vi "MOKE_Teperature and FIeld Sweep_1022D.vi"() -> ()   [LabVIEW 2022 SP3]
uses:
  <vilib>/Analysis/baseanly.llb/Mean (DBL).vi
  <vilib>/Utility/file.llb/Write Delimited Spreadsheet (string).vi
  <vilib>/Utility/file.llb/Write Delimited Spreadsheet (DBL).vi
  <vilib>/Analysis/NI_AALBase.lvlib
panel:
  in  "Read Status":bool
  in  "Wait for position/focus check every (Oe)":i32
  out "Rh1 B/A v F":cluster{dbl[], dbl[]}(graph)
  out "Temperature Status":i32(ring) items=["TemperatureUnknown"=0, "Stable"=1, "Tracking"=2, "Near"=5, "Chasing"=6, "Filling"=7, "Standby"=10, "Disabled"=13, "ImpedanceNotFunction"=14, "TempFailure"=15]
  out "Field Status":i32(ring) items=["MagnetUnknown"=0, "StablePersistent"=1, "WarmingSwitch"=2, "CoolingSwitch"=3, "StableDriven"=4, "Iterating"=5, "Charging"=6, "Discharging"=7, "CurrentError"=8, "MagnetFailure"=15]
  out "Field":dbl
  out "Temperature":dbl
  in  "Initialize":bool
  in  "System Stablization (s)":dbl=0.1 format="%#_13g"
  in  "Low Value (Oe)":dbl=-30000.0
  in  "High Value (Oe)":dbl=30000.0
  in  "Sweep Field Approach":i32(ring) items=["Linear", "NoOvershoot", "Oscillate"]
  in  "Sweep F Rate (Oe/s)":dbl=200.0 format="%#_13g"
  in  "Sweep F mode":i32(ring) items=["Persistent", "Driven"]
  in  "Set Fixed T":dbl=2.0
  in  "Fixed Temperature Approach":i32(ring)=1 items=["FastSettle", "NoOvershoot"]
  in  "FIxed T  Rate (K/min)":dbl=20.0
  out "PhaseA-F":cluster{dbl[], dbl[]}(graph)
  out "RA-F":cluster{dbl[], dbl[]}(graph)
  out "Phaseh1B-F":cluster{dbl[], dbl[]}(graph)
  out "Rh1B-F":cluster{dbl[], dbl[]}(graph)
  out "phase B 2":dbl
  in  "Phase B 2":u16(ring)=3 items=["X", "Y", "R", "Theta", "Frequency", "Noise", "Xh1", "Yh1", "Rh1", "Theta h1", "Xh2", "Yh2", "Rh2", "Theta h2"]
  out "phase A 2":dbl
  in  "Phase A 2":u16(ring)=3 items=["X", "Y", "R", "Theta", "Frequency", "Noise", "Xh1", "Yh1", "Rh1", "Theta h1", "Xh2", "Yh2", "Rh2", "Theta h2"]
  out "para1 Measurement (mV) 2":dbl=1.49013e-07
  in  "F Clear Plot A":bool
  in  "Parameter A 2":u16(ring)=2 items=["X", "Y", "R", "Theta", "Frequency", "Noise", "Xh1", "Yh1", "Rh1", "Theta h1", "Xh2", "Yh2", "Rh2", "Theta h2"]
  out "para2 Measurement (uV) 2":dbl=1.49013e-07
  in  "F Clear Plot B":bool
  in  "Parameter B 2":u16(ring)=2 items=["X", "Y", "R", "Theta", "Frequency", "Noise", "Xh1", "Yh1", "Rh1", "Theta h1", "Xh2", "Yh2", "Rh2", "Theta h2"]
  out "Field Setting":dbl format="%#_13g"
  out "Fixed Temperature":dbl
  out "Measured Field":dbl
  out "Field Status":i32(ring) items=["MagnetUnknown"=0, "StablePersistent"=1, "WarmingSwitch"=2, "CoolingSwitch"=3, "StableDriven"=4, "Iterating"=5, "Charging"=6, "Discharging"=7, "CurrentError"=8, "MagnetFailure"=15]
  out "Temperature Status":i32(ring) items=["TemperatureUnknown"=0, "Stable"=1, "Tracking"=2, "Near"=5, "Chasing"=6, "Filling"=7, "Standby"=10, "Disabled"=13, "ImpedanceNotFunction"=14, "TempFailure"=15]
  out "Measuring F":bool
  in  "Step(Oe)":i32=2000
  out "F loop run":i32
  out "Temperature Status":i32(ring) items=["TemperatureUnknown"=0, "Stable"=1, "Tracking"=2, "Near"=5, "Chasing"=6, "Filling"=7, "Standby"=10, "Disabled"=13, "ImpedanceNotFunction"=14, "TempFailure"=15]
  out "Field Status":i32(ring) items=["MagnetUnknown"=0, "StablePersistent"=1, "WarmingSwitch"=2, "CoolingSwitch"=3, "StableDriven"=4, "Iterating"=5, "Charging"=6, "Discharging"=7, "CurrentError"=8, "MagnetFailure"=15]
  out "Fixed Field":dbl
  out "Measured Temperature":dbl
  in  "Delay(T/F)":dbl=5.0
  in  "Set FIxed F (Oe)":dbl format="%#_13g"
  in  "Fixed Field Approach":i32(ring) items=["Linear", "NoOvershoot", "Oscillate"]
  in  "FIxed F Rate (Oe/s)":dbl=100.0 format="%#_13g"
  in  "Fixed F mode":i32(ring) items=["Persistent", "Driven"]
  in  "Sweep Temperature Approach":i32(ring)=1 items=["FastSettle", "NoOvershoot"]
  in  "Sweep T  Rate (K/min)":dbl=10.0
  in  "Sweep T/F":bool
  in  "Remote":bool=TRUE
  in  "IP Address":string="169.254.170.239"
  out "Measuring T":bool
  in  "A Sine Output Amplitude (V)":sgl=0.1
  in  "path (folder + filename)":string="C:\\Users\\Public\\OneDrive\\Desktop\\MOKE program\\sweep files"
  in  "LOCKIN address":refnum<visa-resource-name>="COM3"
  out "PhaseA-T":cluster{dbl[], dbl[]}(graph)
  out "RA-T":cluster{dbl[], dbl[]}(graph)
  out "Phaseh1-T":cluster{dbl[], dbl[]}(graph)
  out "Rh1B-T":cluster{dbl[], dbl[]}(graph)
  out "phase B":dbl
  in  "Phase B":u16(ring)=9 items=["X", "Y", "R", "Theta", "Frequency", "Noise", "Xh1", "Yh1", "Rh1", "Theta h1", "Xh2", "Yh2", "Rh2", "Theta h2"]
  out "phase A":dbl
  in  "Phase A":u16(ring)=3 items=["X", "Y", "R", "Theta", "Frequency", "Noise", "Xh1", "Yh1", "Rh1", "Theta h1", "Xh2", "Yh2", "Rh2", "Theta h2"]
  out "para1 Measurement (mV)":dbl=1.49013e-07
  in  "T Clear Plot A":bool
  in  "Parameter A":u16(ring)=2 items=["X", "Y", "R", "Theta", "Frequency", "Noise", "Xh1", "Yh1", "Rh1", "Theta h1", "Xh2", "Yh2", "Rh2", "Theta h2"]
  out "para2 Measurement (uV)":dbl=1.49013e-07
  in  "T Clear Plot B":bool
  in  "Parameter B":u16(ring)=8 items=["X", "Y", "R", "Theta", "Frequency", "Noise", "Xh1", "Yh1", "Rh1", "Theta h1", "Xh2", "Yh2", "Rh2", "Theta h2"]
  out "Temperature Setting":dbl format="%#_13g"
  in  "Save data or not":bool=TRUE
  in  "Step(K)":i32=10
  out "T loop run":i32
  in  "B frequency":dbl=267.7 format="%#_13g"
  in  "B Input Connection (0: Single-Ended)":u16(ring)=1 items=["Single-Ended Voltage", "Differential Voltage", "1 MOhm Current Gain", "100 MOhm Current Gain"]
  in  "B harmonic 1":u8=2
  in  "B harmonic 2":u8=3
  in  "B reference Manual Phase":dbl=-59.75
  in  "auto phase B":bool=TRUE
  in  "B Sample time (s)":dbl=0.001 min=0.001 max=100.0 step=0.001
  in  "B Sensitivity":u16(ring)=20 items=["1 nV/fA", "2 nV/fA", "5 nV/fA", "10 nV/fA", "20 nV/fA", "50 nV/fA", "100 nV/fA", "200 nV/fA", "500 nV/fA", "1 uV/pA", "2 uV/pA", "5 uV/pA", "10 uV/pA", "20 uV/pA", "50 uV/pA", "100 uV/pA", "200 uV/pA", "500 uV/pA", "1 mV/nA", "2 mV/nA", "5 mV/nA", "10 mV/nA", "20 mV/nA", "50 mV/nA", "100 mV/nA", "200 mV/nA", "500 mV/nA", "1 V/uA"]
  in  "Enable Sync Filter B (open when f<200Hz)":bool
  in  "B Time Constant":u8(ring)=9 items=["10 us", "30 us", "100 us", "300 us", "1 ms", "3 ms", "10 ms", "30 ms", "100 ms", "300 ms", "1 s", "3 s", "10 s", "30 s", "100 s", "300 s", "1 ks", "3 ks"]
  in  "B Reference Source":u8(ring) items=["External", "Internal", "Internal Sweep", "Channel-A"]
  in  "B Low Pass Filter Slope":u8(ring)=2 items=["6 dB/oct", "12 dB/oct", "18 db/oct", "24 dB/oct"]
  in  "A frequency":dbl=267.7 format="%#_13g"
  in  "A Input Connection (0: Single-Ended)":u16(ring)=1 items=["Single-Ended Voltage", "Differential Voltage", "1 MOhm Current Gain", "100 MOhm Current Gain"]
  in  "A harmonic 1":u8=2
  in  "A harmonic 2":u8=3
  in  "A reference Manual Phase":dbl=-59.75
  in  "auto phase A":bool=TRUE
  in  "A Reference Source":u8(ring)=1 items=["External", "Internal", "Internal Sweep"]
  in  "A Sample time (s)":dbl=0.001 min=0.001 max=100.0 step=0.001
  in  "A Time Constant":u8(ring)=9 items=["10 us", "30 us", "100 us", "300 us", "1 ms", "3 ms", "10 ms", "30 ms", "100 ms", "300 ms", "1 s", "3 s", "10 s", "30 s", "100 s", "300 s", "1 ks", "3 ks"]
  in  "Enable Sync Filter A (open when f<200Hz)":bool
  in  "A Sensitivity":u16(ring)=20 items=["1 nV/fA", "2 nV/fA", "5 nV/fA", "10 nV/fA", "20 nV/fA", "50 nV/fA", "100 nV/fA", "200 nV/fA", "500 nV/fA", "1 uV/pA", "2 uV/pA", "5 uV/pA", "10 uV/pA", "20 uV/pA", "50 uV/pA", "100 uV/pA", "200 uV/pA", "500 uV/pA", "1 mV/nA", "2 mV/nA", "5 mV/nA", "10 mV/nA", "20 mV/nA", "50 mV/nA", "100 mV/nA", "200 mV/nA", "500 mV/nA", "1 V/uA"]
  in  "A Low Pass Filter Slope":u8(ring)=2 items=["6 dB/oct", "12 dB/oct", "18 db/oct", "24 dB/oct"]
  in  "stabilization(S)":dbl=0.1 format="%#_13g"
  in  "High Value (K)":dbl=300.0
  in  "Low Value (K)":dbl=2.0
  in  "loop #":i32=1
  # "Status"
  # "opticool ip addresse: 169.254.170.239"
  # "Lock-in Setting"
  # "Channel A"
  # "Channel B"
  # "Sweep F Mesurement"
  # "Temprature and Field Setting"
  # "Sweep T Mesurement"
  # "Sweep F"
  # "Sweep T"
  # "0 for no checks"
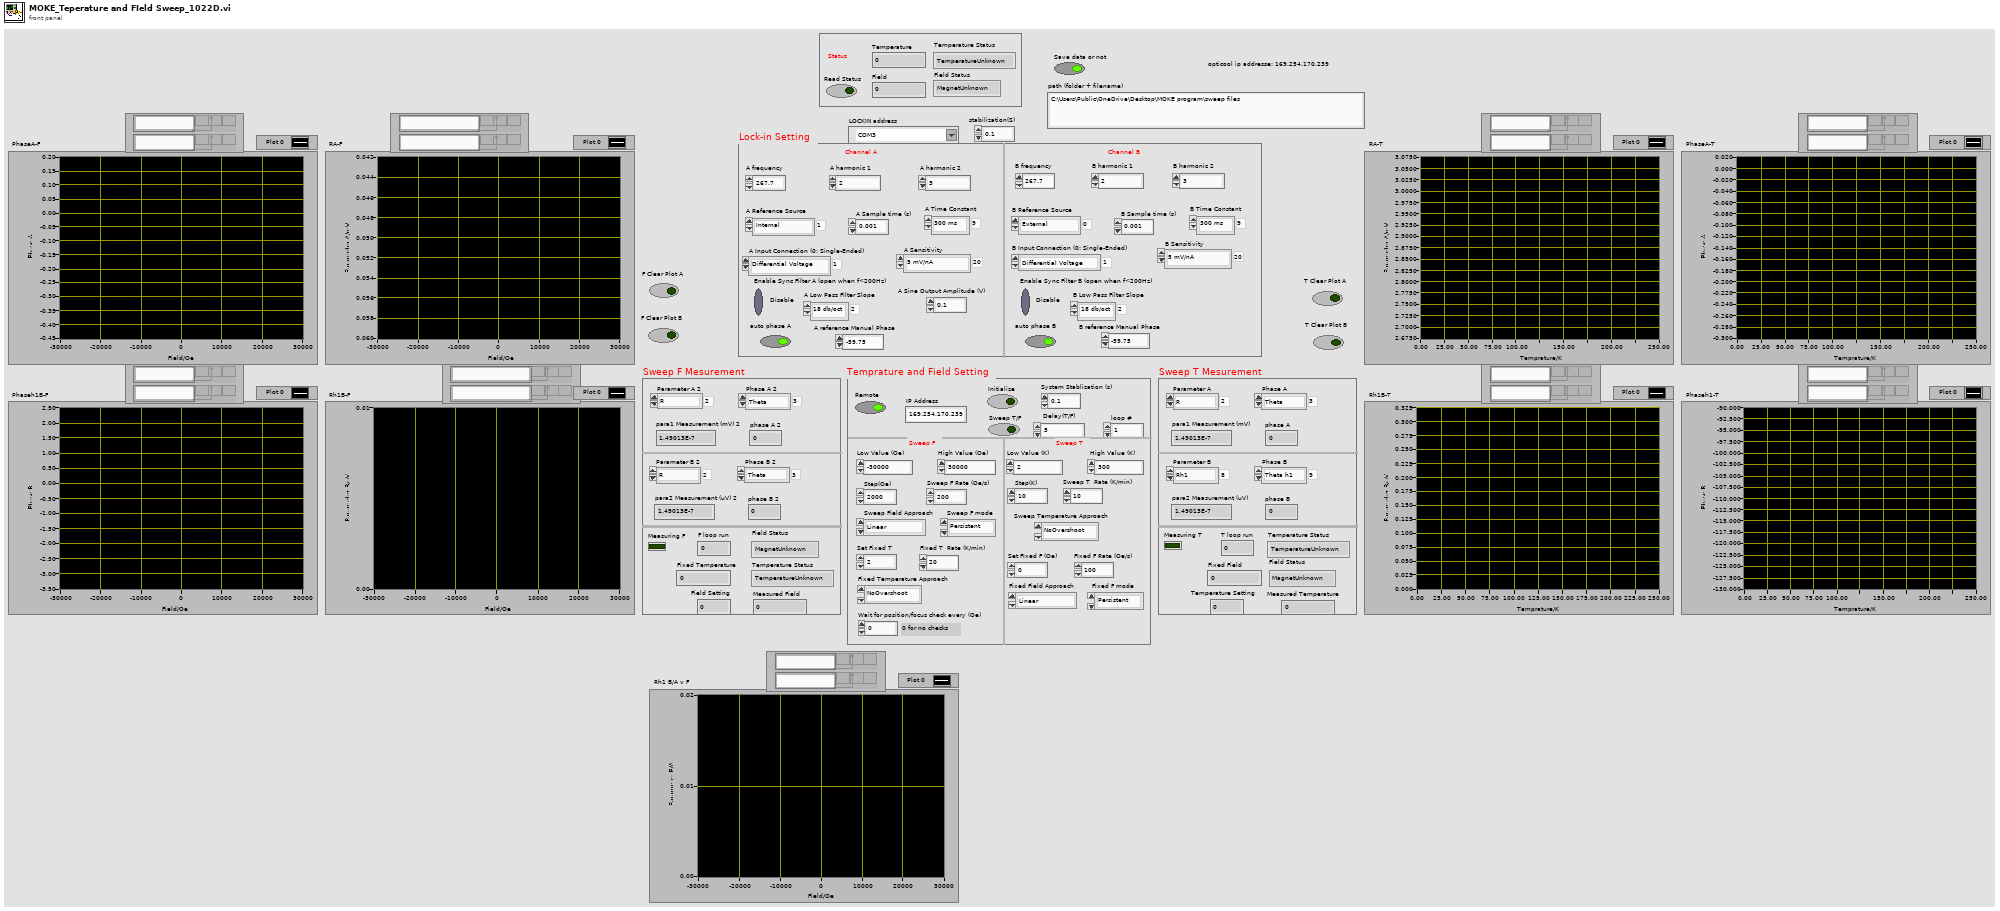
[diagram p1: front panel]
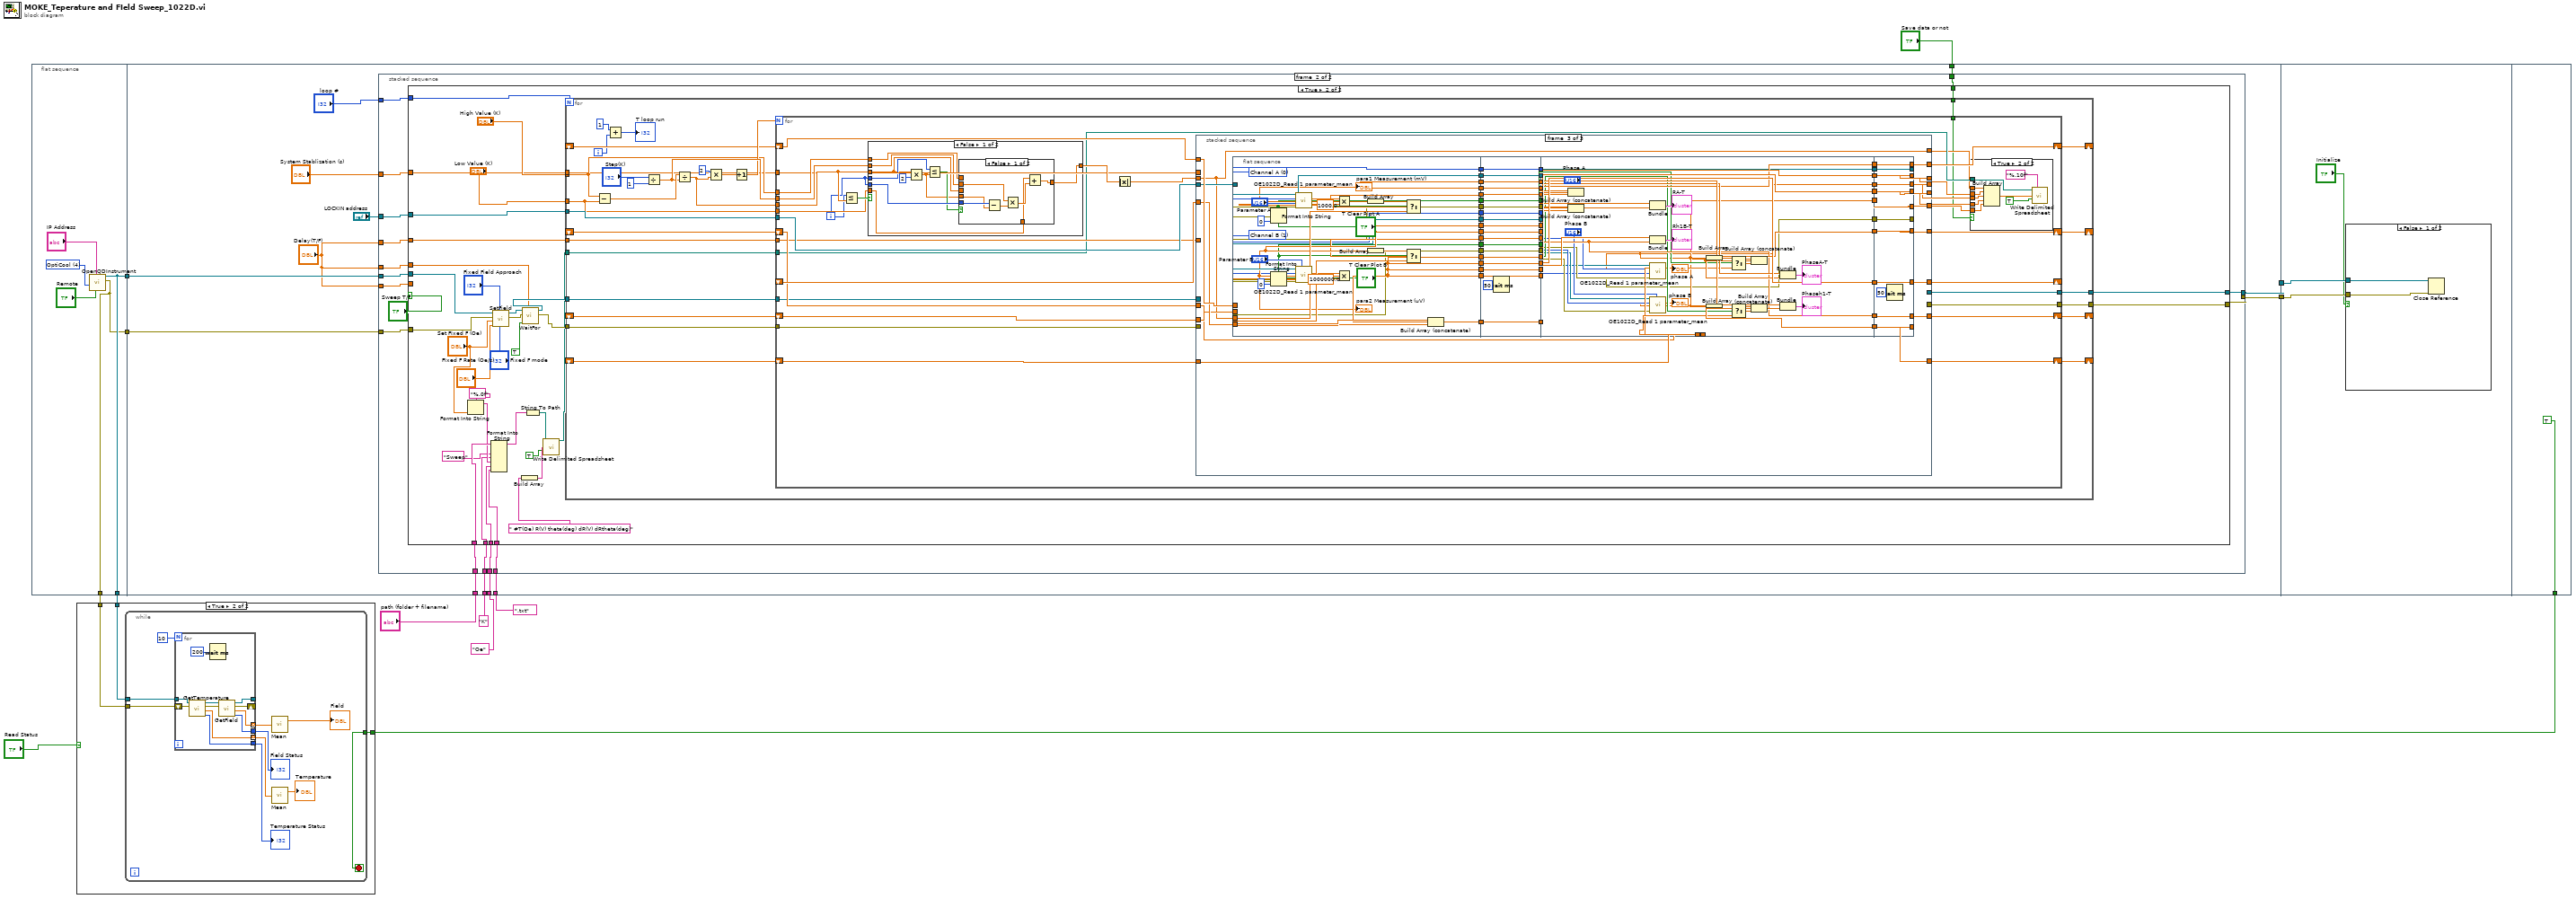
[diagram p0: block diagram]
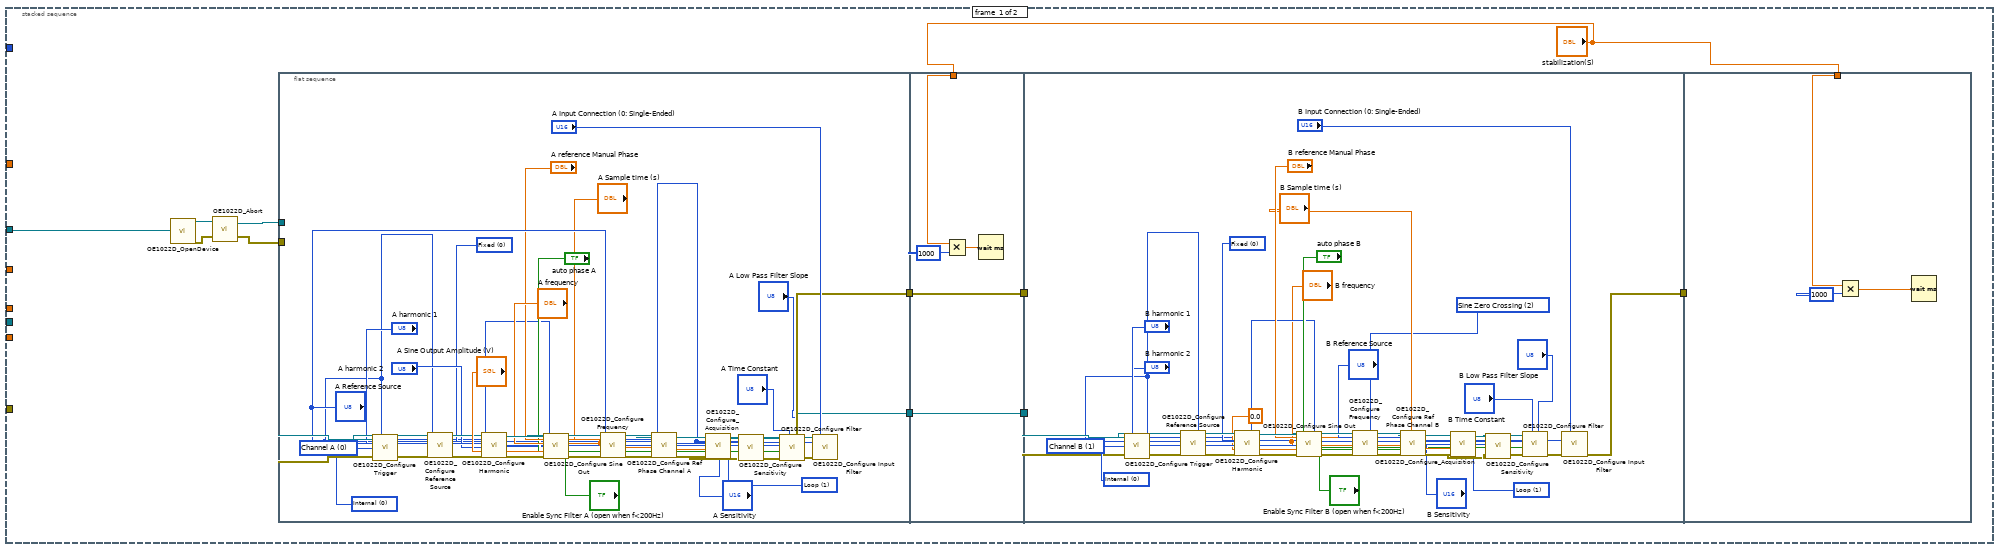
[diagram p3: hidden frame]
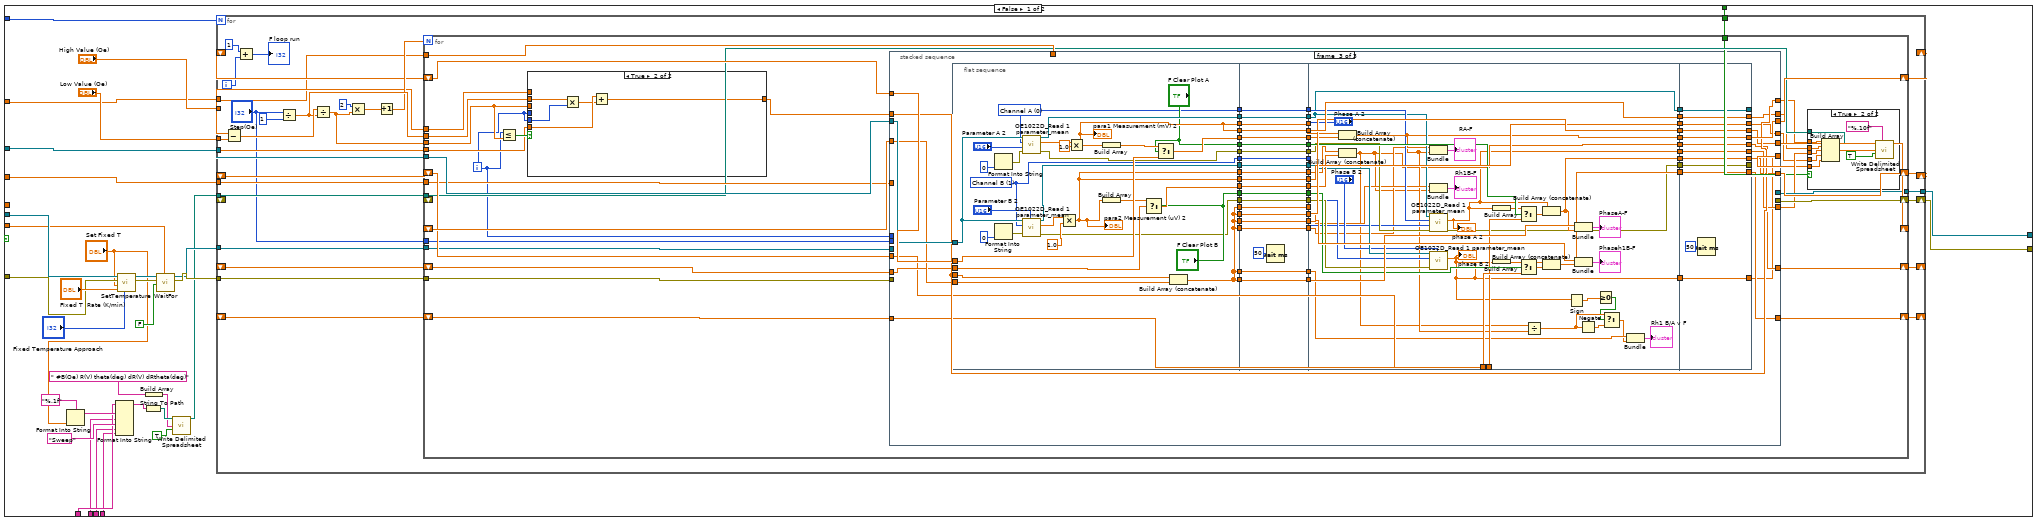
[diagram p4: hidden frame]
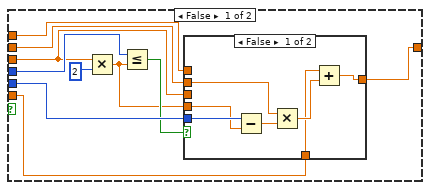
[diagram p6: hidden frame]
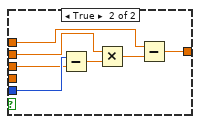
[diagram p7: hidden frame]
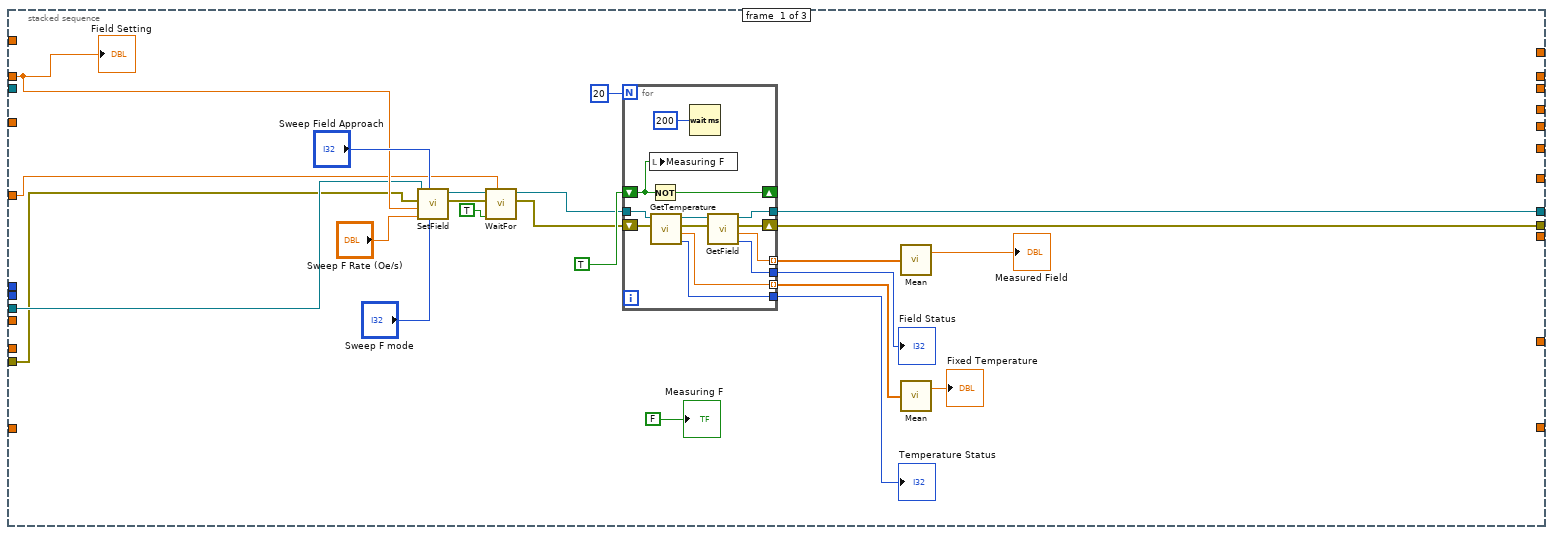
[diagram p8: hidden frame]
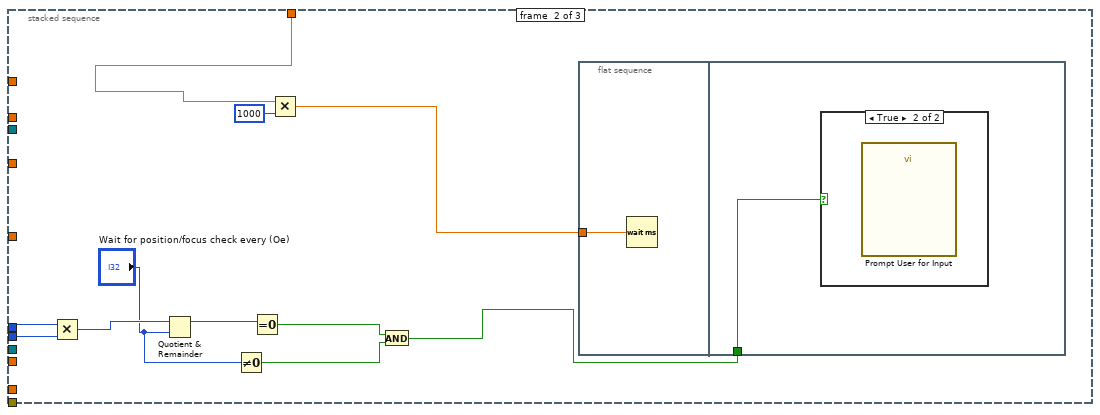
[diagram p9: hidden frame]
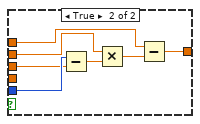
[diagram p12: hidden frame]
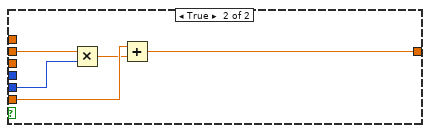
[diagram p13: hidden frame]
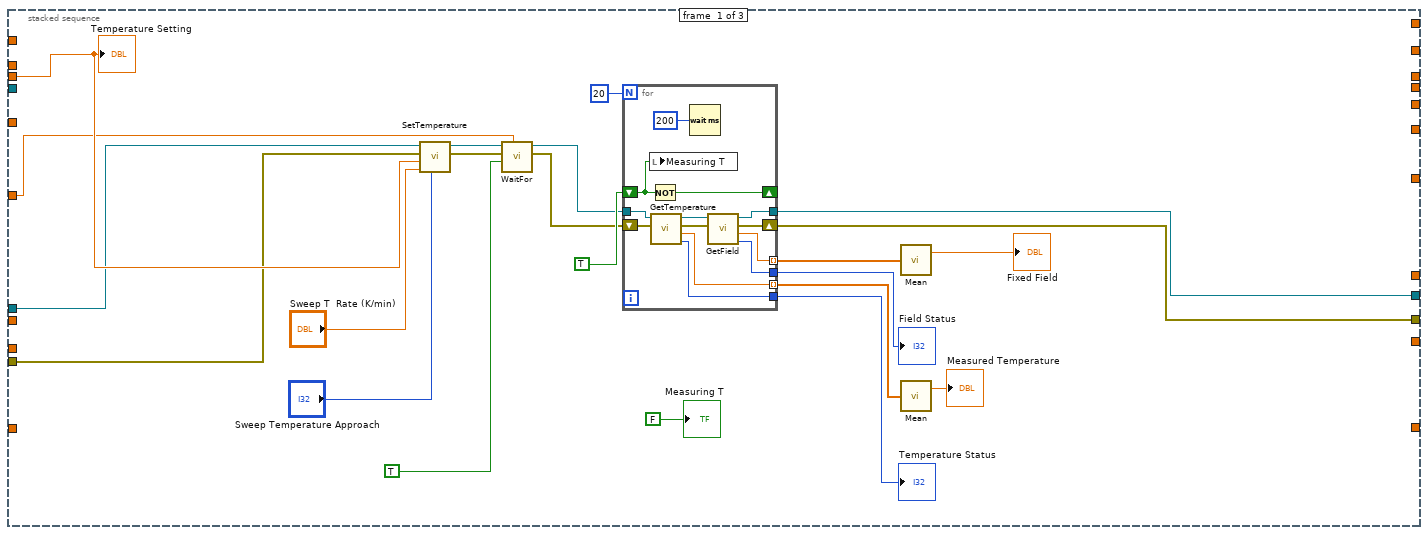
[diagram p14: hidden frame]
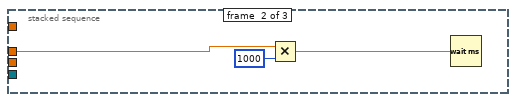
[diagram p15: hidden frame]
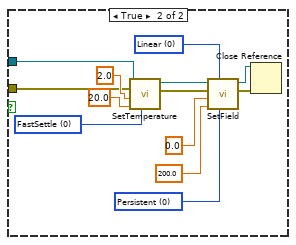
[diagram p16: hidden frame]
diagram:
  n1 = flat-sequence {
    tunnel: [w15] -> w13
    tunnel: [w14] -> w12
    tunnel: [w15] -> w5
    tunnel: [w14] -> w4
    tunnel: w13 -> [w29]
    tunnel: w12 -> [w28]
    tunnel: "path (folder + filename)" -> [w26]
    tunnel: "Oe" -> [w25]
    tunnel: "K" -> [w24]
    tunnel: ".txt" -> [w23]
    tunnel: [w21] -> w7
    tunnel: [w20] -> w6
    tunnel: "Save data or not" -> [w19]
    tunnel: w7 -> [w840]
    tunnel: w6 -> [w839]
    tunnel: [TRUE] -> w2
    frame #0 {
      w16 = 4 items=["PPMS", "VersaLab", "DynaCool", "SVSM", "OptiCool"] ("InstrumentType")
      n2 = call "OpenQDInstrument.vi"("Remote"="Remote", "IP Address"="IP Address", "InstrumentType"=w16) -> ("error out"=w14:errorcluster, "Instrument Ref"=w15:refnum<k24>)  [unwired: 5 in]
    }
    frame #1 {
      n3 = stacked-sequence {
        tunnel: "LOCKIN address" -> [w34 w143]
        tunnel: "loop #" -> [_ w142]
        tunnel: w29 -> [_ w140]
        tunnel: w28 -> [_ w139]
        tunnel: "Delay(T/F)" -> [_ w138]
        tunnel: "Delay(T/F)" -> [_ w137]
        tunnel: "Delay(T/F)" -> [_ w136]
        tunnel: w26 -> [_ w135]
        tunnel: w25 -> [_ w134]
        tunnel: w24 -> [_ w133]
        tunnel: w23 -> [_ w132]
        tunnel: "System Stablization (s)" -> [_ w131]
        tunnel: [_ w130] -> w21
        tunnel: [_ w129] -> w20
        tunnel: w19 -> [_ w128]
        frame #0 {
          n4 = call "OE1022D_OpenDevice.vi"("VISA resource name"=w34) -> ("VISA资源名称输出"=w33:refnum<visa-resource-name>, "错误输出"=w35:errorcluster)  [unwired: 17 in]
          n5 = call "OE1022D_Abort.vi"("error in (no error)"=w35, "VISA resource name"=w33) -> ("error out"=w40:errorcluster, "VISA resource name out"=w41:refnum<visa-resource-name>)
          n6 = flat-sequence {
            tunnel: w41 -> [w81]
            tunnel: [w69] -> w39
            tunnel: w40 -> [w80]
            tunnel: [w57] -> w37
            tunnel: w39 -> [w86]
            tunnel: [w86] -> w38
            tunnel: w37 -> [w85]
            tunnel: [w85] -> w36
            tunnel: "stabilization(S)" -> [w82]
            tunnel: w38 -> [w107]
            tunnel: [w106] -> w42
            tunnel: w36 -> [w105]
            tunnel: w42 -> [_]
            tunnel: "stabilization(S)" -> [w125]
            frame #0 {
              w43 = u8 1 items=["Single", "Loop"] ("Sample Mode (Single/Loop)")
              w56 = u8 0 items=["Fixed", "Linear", "Log"] ("SineOut Mode")
              w58 = u16 0 items=["Internal", "External"] ("Trigger Source (0: Internal)")
              w47 = u8 0 items=["Channel A", "Channel B"] ("OE1022D A/B")
              n7 = call "OE1022D_Configure Trigger.vi"("Trigger Source (0: Internal)"=w58, "error in (no error)   2"=w80, "OE1022D A/B"=w47, "VISA resource name   2"=w81) -> ("error out   2"=w74:errorcluster, "VISA resource name out   2"=w75:refnum<visa-resource-name>)
              n8 = call "OE1022D_Configure Reference Source.vi"("VISA resource name"=w75, "OE1022D A/B"=w47, "Reference Source"="A Reference Source", "error in (no error)"=w74) -> ("VISA resource name out"=w73:refnum<visa-resource-name>, "error out"=w71:errorcluster)  [unwired: 14 in]
              n9 = call "OE1022D_Configure Harmonic.vi"("VISA resource name"=w73, "OE1022D A/B"=w47, "Harmonic 1"="A harmonic 1", "Harmonic 2"="A harmonic 2", "error in (no error)"=w71) -> ("VISA resource name out"=w72:refnum<visa-resource-name>, "error out"=w70:errorcluster)  [unwired: 13 in]
              n10 = call "OE1022D_Configure Sine Out.vi"("VISA resource name"=w72, "SineOut Mode"=w56, "OE1022D A/B"=w47, "Sine Output Amplitude (V)"="A Sine Output Amplitude (V)", "error in (no error)"=w70) -> ("VISA resource name out"=w78:refnum<visa-resource-name>, "error out"=w77:errorcluster)  [unwired: 9 in]
              n11 = call "OE1022D_Configure Frequency.vi"("VISA resource name"=w78, "OE1022D A/B"=w47, "Internal Frequency(Hz)"="A frequency", "error in (no error)"=w77) -> ("VISA resource name out"=w68:refnum<visa-resource-name>, "error out"=w65:errorcluster)  [unwired: 14 in]
              n12 = call "OE1022D_Configure Ref Phase Channel A.vi"("VISA resource name"=w68, "Reference Source"="A Reference Source", "Internal Frequency(Hz)"="A frequency", "Auto Phase (T: Enabled)"="auto phase A", "error in (no error)"=w65, "Manual Phase  (degree)"="A reference Manual Phase") -> ("VISA resource name out"=w67:refnum<visa-resource-name>, "error out"=w66:errorcluster)  [unwired: 12 in]
              n13 = call "OE1022D_Configure_Acquisition.vi"("VISA resource name"=w67, "OE1022D A/B"=w47, "Sample time (s)"="A Sample time (s)", "error in (no error)"=w66, "Sample Mode (Single/Loop)"=w43) -> ("VISA resource name out"=w50:refnum<visa-resource-name>, "error out"=w49:errorcluster)  [unwired: 3 in]
              n14 = call "OE1022D_Configure Sensitivity.vi"("VISA resource name"=w50, "OE1022D A/B"=w47, "Sensitivity"="A Sensitivity", "error in (no error)"=w49) -> ("VISA resource name out"=w54:refnum<visa-resource-name>, "error out"=w53:errorcluster)  [unwired: 14 in]
              n15 = call "OE1022D_Configure Filter.vi"("Low Pass Filter Slope (1: 12dB/oct)"="A Low Pass Filter Slope", "Time Constant (8: 100ms)"="A Time Constant", "error in (no error)"=w53, "Enable Sync Filter (F: Disable)"="Enable Sync Filter A (open when f<200Hz)", "OE1022D A/B"=w47, "VISA resource name"=w54) -> ("error out"=w51:errorcluster, "VISA resource name out"=w52:refnum<visa-resource-name>)  [unwired: 4 in]
              n16 = call "OE1022D_Configure Input Filter.vi"("VISA resource name"=w52, "Input Source"="A Input Connection (0: Single-Ended)", "OE1022D A/B"=w47, "error in (no error)"=w51) -> ("VISA resource name out"=w57:refnum<visa-resource-name>, "error out"=w69:errorcluster)  [unwired: 10 in]
            }
            frame #1 {
              n17 = Multiply(x=w82, y=1000) -> (x*y=w84:dbl)
              n18 = Wait (ms)(milliseconds to wait=w84) -> ()  [unwired: 1 out]
            }
            frame #2 {
              w87 = u8 1 items=["Single", "Loop"] ("Sample Mode (Single/Loop)")
              w89 = u8 2 items=["TTL Pos", "TTL Neg", "Sine Zero Crossing"] ("External Ref Trigger")
              w102 = u8 0 items=["Fixed", "Linear", "Log"] ("SineOut Mode")
              w108 = u16 0 items=["Internal", "External"] ("Trigger Source (0: Internal)")
              w94 = u8 1 items=["Channel A", "Channel B"] ("OE1022D A/B")
              n19 = call "OE1022D_Configure Trigger.vi"("Trigger Source (0: Internal)"=w108, "error in (no error)   2"=w107, "OE1022D A/B"=w94, "VISA resource name   2"=w105) -> ("error out   2"=w120:errorcluster, "VISA resource name out   2"=w121:refnum<visa-resource-name>)
              n20 = call "OE1022D_Configure Reference Source.vi"("VISA resource name"=w121, "OE1022D A/B"=w94, "error in (no error)"=w120) -> ("VISA resource name out"=w119:refnum<visa-resource-name>, "error out"=w117:errorcluster)  [unwired: 15 in]
              n21 = call "OE1022D_Configure Harmonic.vi"("VISA resource name"=w119, "OE1022D A/B"=w94, "Harmonic 1"="B harmonic 1", "Harmonic 2"="B harmonic 2", "error in (no error)"=w117) -> ("VISA resource name out"=w118:refnum<visa-resource-name>, "error out"=w116:errorcluster)  [unwired: 13 in]
              n22 = call "OE1022D_Configure Sine Out.vi"("VISA resource name"=w118, "SineOut Mode"=w102, "OE1022D A/B"=w94, "Sine Output Amplitude (V)"=sgl 0.0, "error in (no error)"=w116) -> ("VISA resource name out"=w123:refnum<visa-resource-name>, "error out"=w122:errorcluster)  [unwired: 9 in]
              n23 = call "OE1022D_Configure Frequency.vi"("VISA resource name"=w123, "OE1022D A/B"=w94, "Internal Frequency(Hz)"="B frequency", "error in (no error)"=w122) -> ("VISA resource name out"=w115:refnum<visa-resource-name>, "error out"=w112:errorcluster)  [unwired: 14 in]
              n24 = call "OE1022D_Configure Ref Phase Channel B.vi"("VISA resource name"=w115, "Reference Source"="B Reference Source", "External Ref Trigger"=w89, "Internal Frequency(Hz)"="B frequency", "Auto Phase (T: Enabled)"="auto phase B", "error in (no error)"=w112, "Manual Phase  (degree)"="B reference Manual Phase") -> ("VISA resource name out"=w114:refnum<visa-resource-name>, "error out"=w113:errorcluster)  [unwired: 11 in]
              n25 = call "OE1022D_Configure_Acquisition.vi"("VISA resource name"=w114, "OE1022D A/B"=w94, "Sample time (s)"="B Sample time (s)", "error in (no error)"=w113, "Sample Mode (Single/Loop)"=w87) -> ("VISA resource name out"=w95:refnum<visa-resource-name>, "error out"=w96:errorcluster)  [unwired: 3 in]
              n26 = call "OE1022D_Configure Sensitivity.vi"("VISA resource name"=w95, "OE1022D A/B"=w94, "Sensitivity"="B Sensitivity", "error in (no error)"=w96) -> ("VISA resource name out"=w99:refnum<visa-resource-name>, "error out"=w98:errorcluster)  [unwired: 14 in]
              n27 = call "OE1022D_Configure Filter.vi"("Low Pass Filter Slope (1: 12dB/oct)"="B Low Pass Filter Slope", "Time Constant (8: 100ms)"="B Time Constant", "error in (no error)"=w98, "Enable Sync Filter (F: Disable)"="Enable Sync Filter B (open when f<200Hz)", "OE1022D A/B"=w94, "VISA resource name"=w99) -> ("error out"=w97:errorcluster)  [unwired: 4 in, 1 out]
              n28 = call "OE1022D_Configure Input Filter.vi"("Input Source"="B Input Connection (0: Single-Ended)", "OE1022D A/B"=w94, "error in (no error)"=w97) -> ("error out"=w106:errorcluster)  [unwired: 11 in, 1 out]
            }
            frame #3 {
              n29 = Multiply(x=w125, y=1000) -> (x*y=w127:dbl)
              n30 = Wait (ms)(milliseconds to wait=w127) -> ()  [unwired: 1 out]
            }
          }
        }
        frame #1 {
          n31 = case shown="True" "Sweep T/F" {
            tunnel: w143 -> [w175 w534]
            tunnel: w142 -> [w176 w533]
            tunnel: w140 -> [w167 w529]
            tunnel: w139 -> [w168 w528]
            tunnel: w138 -> [_ w522]
            tunnel: w137 -> [w174 w521]
            tunnel: w136 -> [w166 _]
            tunnel: w135 -> [w158 w517]
            tunnel: w134 -> [w157 w513]
            tunnel: w133 -> [w156 w514]
            tunnel: w132 -> [w155 w512]
            tunnel: w131 -> [w152 w509]
            tunnel: [w151 w508] -> w130
            tunnel: [w150 w507] -> w129
            tunnel: w128 -> [w149 w506]
            frame False {
              n32 = Format Into String(format string="%.1f", "Set Fixed T") -> (resulting string=w160:string)  [unwired: 2 in, 1 out]
              n33 = Format Into String(initial string=w158, w160, w156, "Sweep", w157, w155) -> (resulting string=w161:string)  [unwired: 2 in, 1 out]
              n34 = call "SetTemperature.vi"("Approach"="Fixed Temperature Approach", "Rate"="FIxed T  Rate (K/min)", "Temperature"="Set Fixed T", "error in (no error)"=w168, "Instrument Ref In"=w167) -> ("error out"=w169:errorcluster, "Instrument Ref Out"=w170:refnum<k24>)  [unwired: 2 in, 1 out]
              n35 = String To Path(string=w161) -> (path=w148:path)
              n36 = Build Array(" #B(Oe) R(V) theta(deg) dR(V) dRtheta(deg)") -> (w146:string[])
              n37 = call "WaitFor.vi"("Delay"=w166, "Wait For Temperature"=FALSE ("WaitForTemperature"), "error in (no error)"=w169, "Instrument Ref In"=w170) -> ("error out"=w165:errorcluster, "Instrument Ref Out"=w164:refnum<k24>)  [unwired: 6 in]
              n38 = call-poly <vilib>:"Write Delimited Spreadsheet.vi"("file path (dialog if empty)"=w148, "1D data"=w146, "append to file? (new file:F)"=TRUE) -> ("new file path (Not A Path if cancelled)"=w145:path)  [unwired: 11 in, 1 out]
              n39 = for {
                N: w176 -> [_]
                tunnel: w175 -> [w206]
                tunnel: "Low Value (Oe)" -> [w201]
                tunnel: "High Value (Oe)" -> [w191]
                tunnel: w145 -> [w200]
                shift-right: [w196] -> _
                shift-left: _ -> [w195]
                shift-right: [w190] -> _
                shift-left: _ -> [w189]
                shift-right: [w188] -> _
                shift-left: _ -> [w187]
                shift-right: [w186] -> _
                shift-left: _ -> [w185]
                tunnel: w164 -> [w184]
                tunnel: w165 -> [w183]
                tunnel: w174 -> [w182]
                tunnel: w152 -> [w181]
                shift-right: [w180] -> w151
                shift-left: _ -> [_]
                tunnel: [w179] -> w150
                tunnel: w149 -> [w178]
                i -> [w193]
                n40 = Subtract(x=w191, y=w201) -> (x-y=w203:dbl)
                n41 = Add(x=1, y=w193) -> (x+y=→"F loop run":i32)
                n42 = Divide(x="Step(Oe)", y=1) -> (x/y=w202:dbl)
                n43 = Divide(x=w203, y=w202) -> (x/y=w199:dbl)
                n44 = Multiply(x=2, y=w199) -> (x*y=w198:dbl)
                n45 = Increment(x=w198) -> (x+1=w197:dbl)
                n46 = for {
                  N: w197 -> [_]
                  tunnel: w206 -> [w238]
                  tunnel: w202 -> [w234]
                  shift-right: [w227] -> w196
                  shift-left: w195 -> [w237]
                  tunnel: w199 -> [w232]
                  tunnel: w201 -> [w235]
                  tunnel: w191 -> [w233]
                  tunnel: w200 -> [w215]
                  shift-right: [w226] -> _
                  shift-left: _ -> [w230]
                  shift-right: [w229] -> w190
                  shift-left: w189 -> [w228]
                  shift-right: [w225] -> w188
                  shift-left: w187 -> [w224]
                  shift-right: [w223] -> w186
                  shift-left: w185 -> [w222]
                  tunnel: w184 -> [w221]
                  tunnel: w183 -> [w220]
                  tunnel: w182 -> [w219]
                  tunnel: w181 -> [w218]
                  shift-right: [w217] -> w180
                  shift-left: _ -> [_]
                  tunnel: [w216] -> w179
                  tunnel: w178 -> [w209]
                  tunnel: "Step(Oe)" -> [w207]
                  i -> [w208]
                  n47 = Less Or Equal?(x=w208, y=w232) -> (x <= y?=w236:bool)
                  n48 = case shown="True" w236 {
                    tunnel: w235 -> [w248 w276]
                    tunnel: w208 -> [w257 w275]
                    tunnel: w234 -> [w256 w274]
                    tunnel: [w254 w272] -> w231
                    tunnel: w233 -> [w255 _]
                    tunnel: w232 -> [w250 _]
                    tunnel: w208 -> [w253 _]
                    frame False {
                      n49 = Multiply(x=w250, y=2) -> (x*y=w249:dbl)
                      n50 = Less Or Equal?(x=w253, y=w249) -> (x <= y?=w251:bool)
                      n51 = case shown="False" w251 {
                        tunnel: w257 -> [w264 w271]
                        tunnel: w256 -> [w262 w269]
                        tunnel: w255 -> [_ w267]
                        tunnel: [w260 w266] -> w254
                        tunnel: w250 -> [_ w265]
                        tunnel: w249 -> [w259 _]
                        tunnel: w248 -> [w258 _]
                        frame False {
                          n52 = Subtract(x=w264, y=w259) -> (x-y=w263:dbl)
                          n53 = Multiply(x=w262, y=w263) -> (x*y=w261:dbl)
                          n54 = Add(x=w258, y=w261) -> (x+y=w260:dbl)
                        }
                        frame True {
                          n55 = Subtract(x=w271, y=w265) -> (x-y=w270:dbl)
                          n56 = Multiply(x=w269, y=w270) -> (x*y=w268:dbl)
                          n57 = Subtract(x=w267, y=w268) -> (x-y=w266:dbl)
                        }
                      }
                    }
                    frame True {
                      n58 = Multiply(x=w274, y=w275) -> (x*y=w273:dbl)
                      n59 = Add(x=w276, y=w273) -> (x+y=w272:dbl)
                    }
                  }
                  n60 = stacked-sequence {
                    tunnel: w238 -> [_ _ w390]
                    tunnel: w231 -> [w282 _ w389]
                    tunnel: w237 -> [_ _ w392]
                    tunnel: [_ _ w391] -> w227
                    tunnel: [_ _ w328] -> w213
                    tunnel: [_ _ w389] -> w214
                    tunnel: [_ _ w388] -> w226
                    tunnel: w230 -> [_ _ w387]
                    tunnel: [_ _ w386] -> w212
                    tunnel: [_ _ w385] -> w229
                    tunnel: w228 -> [_ _ w378]
                    tunnel: [_ _ w384] -> w225
                    tunnel: w224 -> [_ _ w379]
                    tunnel: [_ _ w383] -> w223
                    tunnel: w222 -> [_ _ w382]
                    tunnel: [_ _ w381] -> w210
                    tunnel: [_ _ w380] -> w211
                    tunnel: w221 -> [w281 _ _]
                    tunnel: w220 -> [w280 _ _]
                    tunnel: w219 -> [w279 _ _]
                    tunnel: w218 -> [_ w321 _]
                    tunnel: [w278 _ _] -> w217
                    tunnel: [w277 _ _] -> w216
                    tunnel: w208 -> [_ w320 _]
                    tunnel: w207 -> [_ w319 _]
                    frame #0 {
                      n61 = call "SetField.vi"("Mode"="Sweep F mode", "Approach"="Sweep Field Approach", "Rate"="Sweep F Rate (Oe/s)", "Field"=w282, "error in (no error)"=w280, "Instrument Ref In"=w281) -> ("error out"=w286:errorcluster, "Instrument Ref Out"=w287:refnum<k24>)  [unwired: 1 in, 1 out]
                      n62 = call "WaitFor.vi"("Delay"=w279, "Wait For Field"=TRUE, "error in (no error)"=w286, "Instrument Ref In"=w287) -> ("error out"=w284:errorcluster, "Instrument Ref Out"=w283:refnum<k24>)  [unwired: 6 in]
                      n63 = for {
                        N: 20 -> [_]
                        shift-right: [w312] -> _
                        shift-left: TRUE -> [w310]
                        shift-right: [w307] -> w278
                        shift-left: w284 -> [w309]
                        tunnel: w283 -> [w306]
                        tunnel: [w304] -> w277
                        tunnel: [w301] -> w297
                        tunnel: [w300] -> w296
                        tunnel: [w302] -> w294 mode=indexing
                        tunnel: [w303] -> w295 mode=indexing
                        n64 = local write "Measuring F"(w310) -> ()
                        n65 = Not(x=w310) -> (.not. x?=w312:bool)
                        n66 = call "GetTemperature.vi"("error in (no error)"=w309, "Instrument Ref In"=w306) -> ("Temperature\nStatus"=w300:i32, "Temperature"=w303:dbl, "error out"=w308:errorcluster, "Instrument Ref Out"=w305:refnum<k24>)  [unwired: 3 in, 1 out]
                        n67 = Wait (ms)(milliseconds to wait=u32 200) -> ()  [unwired: 1 out]
                        n68 = call "GetField.vi"("error in (no error)"=w308, "Instrument Ref In"=w305) -> ("Field\nStatus"=w301:i32, "Field"=w302:dbl, "error out"=w307:errorcluster, "Instrument Ref Out"=w304:refnum<k24>)  [unwired: 3 in, 1 out]
                      }
                      "Field Status" <- w297
                      "Temperature Status" <- w296
                      n69 = call-poly <vilib>:"Mean.vi"("X"=w294) -> ("mean"=→"Measured Field":dbl)  [unwired: 1 out]
                      n70 = call-poly <vilib>:"Mean.vi"("X"=w295) -> ("mean"=→"Fixed Temperature":dbl)  [unwired: 1 out]
                      "Field Setting" <- w282
                      "Measuring F" <- FALSE
                    }
                    frame #1 {
                      n71 = Multiply(x=w320, y=w319) -> (x*y=w318:i32)
                      n72 = Quotient & Remainder(x=w318, y="Wait for position/focus check every (Oe)") -> (x-y*floor(x/y)=w317:i32)  [unwired: 1 out]
                      n73 = Not Equal To 0?(x="Wait for position/focus check every (Oe)") -> (x != 0?=w313:bool)
                      n74 = Equal To 0?(x=w317) -> (x = 0?=w316:bool)
                      n75 = Multiply(x=w321, y=1000) -> (x*y=w323:dbl)
                      n76 = And(x=w316, y=w313) -> (x .and. y?=w315:bool)
                      n77 = flat-sequence {
                        tunnel: w323 -> [w324]
                        tunnel: w315 -> [w325]
                        frame #0 {
                          n78 = Wait (ms)(milliseconds to wait=w324) -> ()  [unwired: 1 out]
                        }
                        frame #1 {
                          n79 = case shown="True" w325 {
                            frame False {
                            }
                            frame True {
                              n80 = call "Prompt User for Input"() -> ()  [unwired: 17 in, 3 out]
                            }
                          }
                        }
                      }
                    }
                    frame #2 {
                      n81 = flat-sequence {
                        tunnel: w392 -> [w420]
                        tunnel: w390 -> [w411]
                        tunnel: w389 -> [w419]
                        tunnel: w387 -> [w418]
                        tunnel: w382 -> [w409]
                        tunnel: [w416] -> w377
                        tunnel: [w404] -> w375
                        tunnel: [w393] -> w373
                        tunnel: [w402] -> w371
                        tunnel: [w393] -> w369
                        tunnel: [w393] -> w367
                        tunnel: [w393] -> w365
                        tunnel: [w393] -> w363
                        tunnel: [w404] -> w361
                        tunnel: [w403] -> w359
                        tunnel: [w402] -> w357
                        tunnel: [w401] -> w355
                        tunnel: ["F Clear Plot B"] -> w353
                        tunnel: ["F Clear Plot A"] -> w351
                        tunnel: [w398] -> w349
                        tunnel: [w397] -> w347
                        tunnel: [w396] -> w345
                        tunnel: [w395] -> w343
                        tunnel: [w394] -> w341
                        tunnel: [w393] -> w326
                        tunnel: w377 -> [w443]
                        tunnel: [w443] -> w376
                        tunnel: w375 -> [w442]
                        tunnel: [w442] -> w374
                        tunnel: w373 -> [w441]
                        tunnel: [w441] -> w372
                        tunnel: w371 -> [w440]
                        tunnel: [w440] -> w370
                        tunnel: w369 -> [w439]
                        tunnel: [w439] -> w368
                        tunnel: w367 -> [w438]
                        tunnel: [w438] -> w366
                        tunnel: w365 -> [w437]
                        tunnel: [w437] -> w364
                        tunnel: w363 -> [w436]
                        tunnel: [w436] -> w362
                        tunnel: w361 -> [w435]
                        tunnel: [w435] -> w360
                        tunnel: w359 -> [w434]
                        tunnel: [w434] -> w358
                        tunnel: w357 -> [w433]
                        tunnel: [w433] -> w356
                        tunnel: w355 -> [w432]
                        tunnel: [w432] -> w354
                        tunnel: w353 -> [w431]
                        tunnel: [w431] -> w352
                        tunnel: w351 -> [w430]
                        tunnel: [w430] -> w350
                        tunnel: w349 -> [w429]
                        tunnel: [w429] -> w348
                        tunnel: w347 -> [w428]
                        tunnel: [w428] -> w346
                        tunnel: w345 -> [w427]
                        tunnel: [w427] -> w344
                        tunnel: w343 -> [w426]
                        tunnel: [w426] -> w342
                        tunnel: w341 -> [w425]
                        tunnel: [w425] -> w340
                        tunnel: [w423] -> w327
                        tunnel: w326 -> [w423]
                        tunnel: w376 -> [w459]
                        tunnel: w374 -> [w488]
                        tunnel: w372 -> [w487]
                        tunnel: w370 -> [w486]
                        tunnel: w368 -> [w485]
                        tunnel: w366 -> [w456]
                        tunnel: w364 -> [w455]
                        tunnel: w362 -> [w481]
                        tunnel: w360 -> [w478]
                        tunnel: w358 -> [w477]
                        tunnel: w356 -> [w475]
                        tunnel: w354 -> [w474]
                        tunnel: w379 -> [w473]
                        tunnel: w352 -> [w472]
                        tunnel: w378 -> [w470]
                        tunnel: w350 -> [w469]
                        tunnel: w348 -> [w465]
                        tunnel: w346 -> [w464]
                        tunnel: w344 -> [w463]
                        tunnel: w342 -> [w461]
                        tunnel: w340 -> [w460]
                        tunnel: [w459] -> w339
                        tunnel: [w454] -> w338
                        tunnel: [w488] -> w337
                        tunnel: [w487] -> w336
                        tunnel: [w450] -> w335
                        tunnel: [w458] -> w334
                        tunnel: [w479] -> w333
                        tunnel: [w476] -> w332
                        tunnel: [w453] -> w331
                        tunnel: [w486] -> w330
                        tunnel: [w446] -> w329
                        tunnel: w327 -> [w452]
                        tunnel: [w490] -> w380
                        tunnel: [w491] -> w381
                        tunnel: [w492] -> w383
                        tunnel: [w493] -> w384
                        tunnel: [w494] -> w385
                        tunnel: [w495] -> _
                        tunnel: [w496] -> w386
                        tunnel: [w497] -> w388
                        tunnel: [w498] -> w328
                        tunnel: [w499] -> w391
                        tunnel: [w500] -> _
                        tunnel: w339 -> [w500]
                        tunnel: w338 -> [w499]
                        tunnel: w337 -> [w498]
                        tunnel: w336 -> [w497]
                        tunnel: w335 -> [w496]
                        tunnel: w334 -> [w495]
                        tunnel: w333 -> [w494]
                        tunnel: w332 -> [w493]
                        tunnel: w331 -> [w492]
                        tunnel: w330 -> [w491]
                        tunnel: w329 -> [w490]
                        frame #0 {
                          w397 = u8 1 items=["Channel A", "Channel B"] ("Channel A/B for Parameter1")
                          w394 = u8 0 items=["Channel A", "Channel B"] ("Channel A/B for Parameter1")
                          n82 = Format Into String(0) -> (error out=w417:errorcluster)  [unwired: 3 in, 1 out]
                          n83 = Format Into String(0) -> (error out=w412:errorcluster)  [unwired: 3 in, 1 out]
                          n84 = call "OE1022D_Read 1 parameter_mean.vi"("错误输入（无错误）"=w417, "Parameter"="Parameter A 2", "Channel (0: A)"=w394, "VISA resource name"=w411) -> ("error out"=w395:errorcluster, "Measurement"=w406:dbl, "VISA resource name out"=w416:refnum<visa-resource-name>)  [unwired: 5 in]
                          n85 = call "OE1022D_Read 1 parameter_mean.vi"("Parameter 2"="Parameter B 2", "错误输入（无错误）"=w412, "Channel (0: A)"=w397, "VISA resource name"=w411) -> ("error out"=w398:errorcluster, "Measurement"=w405:dbl, "VISA resource name out"=w396:refnum<visa-resource-name>)  [unwired: 5 in]
                          n86 = Multiply(x=w405, y=1.0) -> (x*y=w402:dbl)
                          "para2 Measurement (uV) 2" <- w402
                          n87 = Multiply(x=w406, y=1.0) -> (x*y=w404:dbl)
                          "para1 Measurement (mV) 2" <- w404
                          n88 = Build Array(w404) -> (w421:dbl[])
                          n89 = Build Array(w402) -> (w413:dbl[])
                          n90 = Select(t=w413, s="F Clear Plot B", f=w409) -> (s? t:f=w401:dbl[])
                          n91 = Select(t=w421, s="F Clear Plot A", f=w420) -> (s? t:f=w403:dbl[])
                          n92 = Build Array (concatenate)(w419, w418) -> (w393:dbl[])
                        }
                        frame #1 {
                          n93 = Wait (ms)(milliseconds to wait=u32 50) -> ()  [unwired: 1 out]
                        }
                        frame #2 {
                          n94 = Build Array (concatenate)(w478, w477) -> (w454:dbl[])
                          n95 = Build Array (concatenate)(w475, w474) -> (w453:dbl[])
                          n96 = Bundle(w455, w454) -> (→"RA-F":cluster{dbl[], dbl[]})  [unwired: 1 in]
                          n97 = Bundle(w456, w453) -> (→"Rh1B-F":cluster{dbl[], dbl[]})  [unwired: 1 in]
                          n98 = call "OE1022D_Read 1 parameter_mean.vi"("错误输入（无错误）"=w461, "Parameter"="Phase A 2", "Channel (0: A)"=w460, "VISA resource name"=w459) -> ("error out"=w458:errorcluster, "Measurement"=w450:dbl)  [unwired: 5 in, 1 out]
                          "phase A 2" <- w450
                          n99 = call "OE1022D_Read 1 parameter_mean.vi"("Parameter 2"="Phase B 2", "错误输入（无错误）"=w465, "Channel (0: A)"=w464, "VISA resource name"=w463) -> ("Measurement"=w446:dbl)  [unwired: 5 in, 2 out]
                          "phase B 2" <- w446
                          n100 = Build Array(w450) -> (w466:dbl[])
                          n101 = Build Array(w446) -> (w467:dbl[])
                          n102 = Select(t=w466, s=w469, f=w470) -> (s? t:f=w468:dbl[])
                          n103 = Select(t=w467, s=w472, f=w473) -> (s? t:f=w471:dbl[])
                          n104 = Divide(x=w453, y=w454) -> (x/y=w447:dbl[])
                          n105 = Build Array (concatenate)(w450, w468) -> (w479:dbl[])
                          n106 = Build Array (concatenate)(w446, w471) -> (w476:dbl[])
                          n107 = Sign(1:w446) -> (0:w444:dbl)
                          n108 = Bundle(w481, w479) -> (→"PhaseA-F":cluster{dbl[], dbl[]})  [unwired: 1 in]
                          n109 = Bundle(w485, w476) -> (→"Phaseh1B-F":cluster{dbl[], dbl[]})  [unwired: 1 in]
                          n110 = Negate(x=w447) -> (-x=w448:dbl[])
                          n111 = Greater Or Equal To 0?(x=w444) -> (x >= 0?=w445:bool)
                          n112 = Select(t=w447, s=w445, f=w448) -> (s? t:f=w449:dbl[])
                          n113 = Bundle(w452, w449) -> (→"Rh1 B/A v F":cluster{dbl[], dbl[]})  [unwired: 1 in]
                        }
                        frame #3 {
                          n114 = Wait (ms)(milliseconds to wait=u32 50) -> ()  [unwired: 1 out]
                        }
                      }
                    }
                  }
                  n115 = case shown="True" w209 {
                    tunnel: w213 -> [_ w242]
                    tunnel: w214 -> [_ w247]
                    tunnel: w215 -> [_ w245]
                    tunnel: w212 -> [_ w241]
                    tunnel: w210 -> [_ w240]
                    tunnel: w211 -> [_ w239]
                    frame False {
                    }
                    frame True {
                      n116 = Build Array(w247, w242, w241, w240, w239) -> (w244:dbl[])
                      n117 = call-poly <vilib>:"Write Delimited Spreadsheet.vi"("file path (dialog if empty)"=w245, "format (%.3f)"="%.10f", "1D data"=w244, "append to file? (new file:F)"=TRUE) -> ()  [unwired: 10 in, 2 out]
                    }
                  }
                }
              }
            }
            frame True {
              n118 = Format Into String(format string="%.0f", "Set FIxed F (Oe)") -> (resulting string=w516:string)  [unwired: 2 in, 1 out]
              n119 = Format Into String(initial string=w517, "Sweep", w514, w516, w513, w512) -> (resulting string=w518:string)  [unwired: 2 in, 1 out]
              n120 = call "SetField.vi"("Mode"="Fixed F mode", "Approach"="Fixed Field Approach", "Rate"="FIxed F Rate (Oe/s)", "Field"="Set FIxed F (Oe)", "error in (no error)"=w528, "Instrument Ref In"=w529) -> ("error out"=w524:errorcluster, "Instrument Ref Out"=w526:refnum<k24>)  [unwired: 1 in, 1 out]
              n121 = Build Array(" #T(Oe) R(V) theta(deg) dR(V) dRtheta(deg)") -> (w505:string[])
              n122 = call "WaitFor.vi"("Delay"=w522, "Wait For Field"=TRUE, "error in (no error)"=w524, "Instrument Ref In"=w526) -> ("error out"=w525:errorcluster, "Instrument Ref Out"=w527:refnum<k24>)  [unwired: 6 in]
              n123 = String To Path(string=w518) -> (path=w502:path)
              n124 = call-poly <vilib>:"Write Delimited Spreadsheet.vi"("file path (dialog if empty)"=w502, "1D data"=w505, "append to file? (new file:F)"=TRUE) -> ("new file path (Not A Path if cancelled)"=w501:path)  [unwired: 11 in, 1 out]
              n125 = for {
                N: w533 -> [_]
                tunnel: w534 -> [w564]
                tunnel: "Low Value (K)" -> [w558]
                tunnel: "High Value (K)" -> [w548]
                tunnel: w501 -> [w557]
                shift-right: [w553] -> _
                shift-left: _ -> [w552]
                shift-right: [w547] -> _
                shift-left: _ -> [w546]
                shift-right: [w545] -> _
                shift-left: _ -> [w544]
                shift-right: [w543] -> _
                shift-left: _ -> [w542]
                tunnel: w527 -> [w541]
                tunnel: w525 -> [w540]
                tunnel: w521 -> [w539]
                tunnel: w509 -> [w538]
                tunnel: [w537] -> w508
                tunnel: [w536] -> w507
                tunnel: w506 -> [w535]
                i -> [w550]
                n126 = Subtract(x=w548, y=w558) -> (x-y=w560:dbl)
                n127 = Add(x=1, y=w550) -> (x+y=→"T loop run":i32)
                n128 = Divide(x="Step(K)", y=1) -> (x/y=w559:dbl)
                n129 = Divide(x=w560, y=w559) -> (x/y=w556:dbl)
                n130 = Multiply(x=2, y=w556) -> (x*y=w555:dbl)
                n131 = Increment(x=w555) -> (x+1=w554:dbl)
                n132 = for {
                  N: w554 -> [_]
                  tunnel: w564 -> [w596]
                  tunnel: w559 -> [w592]
                  shift-right: [w583] -> w553
                  shift-left: w552 -> [w595]
                  tunnel: w556 -> [w590]
                  tunnel: w558 -> [w593]
                  tunnel: w548 -> [w591]
                  tunnel: w557 -> [w567]
                  shift-right: [w572] -> _
                  shift-left: _ -> [w586]
                  shift-right: [w585] -> w547
                  shift-left: w546 -> [w584]
                  shift-right: [w582] -> w545
                  shift-left: w544 -> [w581]
                  shift-right: [w580] -> w543
                  shift-left: w542 -> [w579]
                  tunnel: w541 -> [w578]
                  tunnel: w540 -> [w577]
                  tunnel: w539 -> [w576]
                  tunnel: w538 -> [w575]
                  tunnel: [w574] -> w537
                  tunnel: [w573] -> w536
                  tunnel: w535 -> [w565]
                  i -> [w589]
                  n133 = Less Or Equal?(x=w589, y=w590) -> (x <= y?=w594:bool)
                  n134 = case shown="False" w594 {
                    tunnel: w593 -> [w606 w634]
                    tunnel: w589 -> [w615 w633]
                    tunnel: w592 -> [w614 w632]
                    tunnel: [w612 w630] -> w588
                    tunnel: w591 -> [w613 _]
                    tunnel: w590 -> [w608 _]
                    tunnel: w589 -> [w611 _]
                    frame False {
                      n135 = Multiply(x=w608, y=2) -> (x*y=w607:dbl)
                      n136 = Less Or Equal?(x=w611, y=w607) -> (x <= y?=w609:bool)
                      n137 = case shown="False" w609 {
                        tunnel: w615 -> [w622 w629]
                        tunnel: w614 -> [w620 w627]
                        tunnel: w613 -> [_ w625]
                        tunnel: [w618 w624] -> w612
                        tunnel: w608 -> [_ w623]
                        tunnel: w607 -> [w617 _]
                        tunnel: w606 -> [w616 _]
                        frame False {
                          n138 = Subtract(x=w622, y=w617) -> (x-y=w621:dbl)
                          n139 = Multiply(x=w620, y=w621) -> (x*y=w619:dbl)
                          n140 = Add(x=w616, y=w619) -> (x+y=w618:dbl)
                        }
                        frame True {
                          n141 = Subtract(x=w629, y=w623) -> (x-y=w628:dbl)
                          n142 = Multiply(x=w627, y=w628) -> (x*y=w626:dbl)
                          n143 = Subtract(x=w625, y=w626) -> (x-y=w624:dbl)
                        }
                      }
                    }
                    frame True {
                      n144 = Multiply(x=w632, y=w633) -> (x*y=w631:dbl)
                      n145 = Add(x=w634, y=w631) -> (x+y=w630:dbl)
                    }
                  }
                  n146 = Absolute Value(x=w588) -> (abs(x)=w587:dbl)
                  n147 = stacked-sequence {
                    tunnel: w596 -> [_ _ w735]
                    tunnel: w587 -> [w653 _ w673]
                    tunnel: w595 -> [_ _ w737]
                    tunnel: [_ _ w736] -> w583
                    tunnel: [_ _ w734] -> w568
                    tunnel: [_ _ w733] -> w572
                    tunnel: w586 -> [_ _ w732]
                    tunnel: [_ _ w731] -> w569
                    tunnel: [_ _ w730] -> w585
                    tunnel: w584 -> [_ _ w724]
                    tunnel: [_ _ w729] -> w582
                    tunnel: w581 -> [_ _ w725]
                    tunnel: [_ _ w728] -> w580
                    tunnel: w579 -> [_ _ w727]
                    tunnel: [_ _ w674] -> w570
                    tunnel: [_ _ w726] -> w571
                    tunnel: w578 -> [w652 _ _]
                    tunnel: w577 -> [w651 _ _]
                    tunnel: w576 -> [w648 _ _]
                    tunnel: w575 -> [_ w670 _]
                    tunnel: [w636 _ _] -> w574
                    tunnel: [w635 _ _] -> w573
                    tunnel: [_ _ w673] -> w566
                    frame #0 {
                      n148 = call "SetTemperature.vi"("Approach"="Sweep Temperature Approach", "Rate"="Sweep T  Rate (K/min)", "Temperature"=w653, "error in (no error)"=w651, "Instrument Ref In"=w652) -> ("error out"=w649:errorcluster, "Instrument Ref Out"=w650:refnum<k24>)  [unwired: 2 in, 1 out]
                      n149 = call "WaitFor.vi"("Delay"=w648, "Wait For Temperature"=TRUE ("WaitForTemperature"), "error in (no error)"=w649, "Instrument Ref In"=w650) -> ("error out"=w639:errorcluster, "Instrument Ref Out"=w638:refnum<k24>)  [unwired: 6 in]
                      n150 = for {
                        N: 20 -> [_]
                        shift-right: [w669] -> _
                        shift-left: TRUE -> [w667]
                        shift-right: [w664] -> w636
                        shift-left: w639 -> [w666]
                        tunnel: w638 -> [w663]
                        tunnel: [w661] -> w635
                        tunnel: [w658] -> w645
                        tunnel: [w657] -> w644
                        tunnel: [w659] -> w642 mode=indexing
                        tunnel: [w660] -> w643 mode=indexing
                        n151 = local write "Measuring T"(w667) -> ()
                        n152 = Not(x=w667) -> (.not. x?=w669:bool)
                        n153 = call "GetTemperature.vi"("error in (no error)"=w666, "Instrument Ref In"=w663) -> ("Temperature\nStatus"=w657:i32, "Temperature"=w660:dbl, "error out"=w665:errorcluster, "Instrument Ref Out"=w662:refnum<k24>)  [unwired: 3 in, 1 out]
                        n154 = Wait (ms)(milliseconds to wait=u32 200) -> ()  [unwired: 1 out]
                        n155 = call "GetField.vi"("error in (no error)"=w665, "Instrument Ref In"=w662) -> ("Field\nStatus"=w658:i32, "Field"=w659:dbl, "error out"=w664:errorcluster, "Instrument Ref Out"=w661:refnum<k24>)  [unwired: 3 in, 1 out]
                      }
                      "Field Status" <- w645
                      "Temperature Status" <- w644
                      n156 = call-poly <vilib>:"Mean.vi"("X"=w642) -> ("mean"=→"Fixed Field":dbl)  [unwired: 1 out]
                      n157 = call-poly <vilib>:"Mean.vi"("X"=w643) -> ("mean"=→"Measured Temperature":dbl)  [unwired: 1 out]
                      "Temperature Setting" <- w653
                      "Measuring T" <- FALSE
                    }
                    frame #1 {
                      n158 = Multiply(x=w670, y=1000) -> (x*y=w672:dbl)
                      n159 = Wait (ms)(milliseconds to wait=w672) -> ()  [unwired: 1 out]
                    }
                    frame #2 {
                      n160 = flat-sequence {
                        tunnel: w737 -> [w765]
                        tunnel: w735 -> [w756]
                        tunnel: w673 -> [w764]
                        tunnel: w732 -> [w763]
                        tunnel: w727 -> [w754]
                        tunnel: [w761] -> w723
                        tunnel: [w748] -> w721
                        tunnel: [w749] -> w719
                        tunnel: [w746] -> w717
                        tunnel: [w749] -> w715
                        tunnel: [w749] -> w713
                        tunnel: [w749] -> w711
                        tunnel: [w749] -> w709
                        tunnel: [w748] -> w707
                        tunnel: [w747] -> w705
                        tunnel: [w746] -> w703
                        tunnel: [w745] -> w701
                        tunnel: ["T Clear Plot B"] -> w699
                        tunnel: ["T Clear Plot A"] -> w697
                        tunnel: [w742] -> w695
                        tunnel: [w741] -> w693
                        tunnel: [w740] -> w691
                        tunnel: [w739] -> w689
                        tunnel: [w738] -> w687
                        tunnel: w723 -> [w787]
                        tunnel: [w787] -> w722
                        tunnel: w721 -> [w786]
                        tunnel: [w786] -> w720
                        tunnel: w719 -> [w785]
                        tunnel: [w785] -> w718
                        tunnel: w717 -> [w784]
                        tunnel: [w784] -> w716
                        tunnel: w715 -> [w783]
                        tunnel: [w783] -> w714
                        tunnel: w713 -> [w782]
                        tunnel: [w782] -> w712
                        tunnel: w711 -> [w781]
                        tunnel: [w781] -> w710
                        tunnel: w709 -> [w780]
                        tunnel: [w780] -> w708
                        tunnel: w707 -> [w779]
                        tunnel: [w779] -> w706
                        tunnel: w705 -> [w778]
                        tunnel: [w778] -> w704
                        tunnel: w703 -> [w777]
                        tunnel: [w777] -> w702
                        tunnel: w701 -> [w776]
                        tunnel: [w776] -> w700
                        tunnel: w699 -> [w775]
                        tunnel: [w775] -> w698
                        tunnel: w697 -> [w774]
                        tunnel: [w774] -> w696
                        tunnel: w695 -> [w773]
                        tunnel: [w773] -> w694
                        tunnel: w693 -> [w772]
                        tunnel: [w772] -> w692
                        tunnel: w691 -> [w771]
                        tunnel: [w771] -> w690
                        tunnel: w689 -> [w770]
                        tunnel: [w770] -> w688
                        tunnel: w687 -> [w769]
                        tunnel: [w769] -> w686
                        tunnel: w722 -> [w791]
                        tunnel: w720 -> [w825]
                        tunnel: w718 -> [w824]
                        tunnel: w716 -> [w823]
                        tunnel: w714 -> [w822]
                        tunnel: w712 -> [w820]
                        tunnel: w710 -> [w818]
                        tunnel: w708 -> [w816]
                        tunnel: w706 -> [w813]
                        tunnel: w704 -> [w812]
                        tunnel: w702 -> [w809]
                        tunnel: w700 -> [w808]
                        tunnel: w725 -> [w806]
                        tunnel: w698 -> [w805]
                        tunnel: w724 -> [w803]
                        tunnel: w696 -> [w802]
                        tunnel: w694 -> [w798]
                        tunnel: w692 -> [w797]
                        tunnel: w690 -> [w796]
                        tunnel: w688 -> [w793]
                        tunnel: w686 -> [w792]
                        tunnel: [w791] -> w685
                        tunnel: [w811] -> w684
                        tunnel: [w825] -> w683
                        tunnel: [w824] -> w682
                        tunnel: [w789] -> w681
                        tunnel: [w790] -> w680
                        tunnel: [w814] -> w679
                        tunnel: [w810] -> w678
                        tunnel: [w807] -> w677
                        tunnel: [w823] -> w676
                        tunnel: [w795] -> w675
                        tunnel: [w829] -> w726
                        tunnel: [w830] -> w674
                        tunnel: [w827] -> w728
                        tunnel: [w831] -> w729
                        tunnel: [w832] -> w730
                        tunnel: [w833] -> _
                        tunnel: [w834] -> w731
                        tunnel: [w835] -> w733
                        tunnel: [w836] -> w734
                        tunnel: [w826] -> w736
                        tunnel: [w837] -> _
                        tunnel: w685 -> [w837]
                        tunnel: w684 -> [w826]
                        tunnel: w683 -> [w836]
                        tunnel: w682 -> [w835]
                        tunnel: w681 -> [w834]
                        tunnel: w680 -> [w833]
                        tunnel: w679 -> [w832]
                        tunnel: w678 -> [w831]
                        tunnel: w677 -> [w827]
                        tunnel: w676 -> [w830]
                        tunnel: w675 -> [w829]
                        frame #0 {
                          w741 = u8 1 items=["Channel A", "Channel B"] ("Channel A/B for Parameter1")
                          w738 = u8 0 items=["Channel A", "Channel B"] ("Channel A/B for Parameter1")
                          n161 = Format Into String(0) -> (error out=w762:errorcluster)  [unwired: 3 in, 1 out]
                          n162 = Format Into String(0) -> (error out=w757:errorcluster)  [unwired: 3 in, 1 out]
                          n163 = call "OE1022D_Read 1 parameter_mean.vi"("错误输入（无错误）"=w762, "Parameter"="Parameter A", "Channel (0: A)"=w738, "VISA resource name"=w756) -> ("error out"=w739:errorcluster, "Measurement"=w751:dbl, "VISA resource name out"=w761:refnum<visa-resource-name>)  [unwired: 5 in]
                          n164 = call "OE1022D_Read 1 parameter_mean.vi"("Parameter 2"="Parameter B", "错误输入（无错误）"=w757, "Channel (0: A)"=w741, "VISA resource name"=w756) -> ("error out"=w742:errorcluster, "Measurement"=w750:dbl, "VISA resource name out"=w740:refnum<visa-resource-name>)  [unwired: 5 in]
                          n165 = Multiply(x=w751, y=1000.0) -> (x*y=w748:dbl)
                          "para1 Measurement (mV)" <- w748
                          n166 = Multiply(x=w750, y=1000000.0) -> (x*y=w746:dbl)
                          "para2 Measurement (uV)" <- w746
                          n167 = Build Array(w748) -> (w766:dbl[])
                          n168 = Build Array(w746) -> (w758:dbl[])
                          n169 = Select(t=w766, s="T Clear Plot A", f=w765) -> (s? t:f=w747:dbl[])
                          n170 = Select(t=w758, s="T Clear Plot B", f=w754) -> (s? t:f=w745:dbl[])
                          n171 = Build Array (concatenate)(w764, w763) -> (w749:dbl[])
                        }
                        frame #1 {
                          n172 = Wait (ms)(milliseconds to wait=u32 50) -> ()  [unwired: 1 out]
                        }
                        frame #2 {
                          n173 = Build Array (concatenate)(w813, w812) -> (w811:dbl[])
                          n174 = Build Array (concatenate)(w809, w808) -> (w807:dbl[])
                          n175 = Bundle(w818, w811) -> (→"RA-T":cluster{dbl[], dbl[]})  [unwired: 1 in]
                          n176 = Bundle(w820, w807) -> (→"Rh1B-T":cluster{dbl[], dbl[]})  [unwired: 1 in]
                          n177 = call "OE1022D_Read 1 parameter_mean.vi"("错误输入（无错误）"=w793, "Parameter"="Phase A", "Channel (0: A)"=w792, "VISA resource name"=w791) -> ("error out"=w790:errorcluster, "Measurement"=w789:dbl)  [unwired: 5 in, 1 out]
                          "phase A" <- w789
                          n178 = call "OE1022D_Read 1 parameter_mean.vi"("Parameter 2"="Phase B", "错误输入（无错误）"=w798, "Channel (0: A)"=w797, "VISA resource name"=w796) -> ("Measurement"=w795:dbl)  [unwired: 5 in, 2 out]
                          "phase B" <- w795
                          n179 = Build Array(w789) -> (w799:dbl[])
                          n180 = Build Array(w795) -> (w800:dbl[])
                          n181 = Select(t=w799, s=w802, f=w803) -> (s? t:f=w801:dbl[])
                          n182 = Select(t=w800, s=w805, f=w806) -> (s? t:f=w804:dbl[])
                          n183 = Build Array (concatenate)(w789, w801) -> (w814:dbl[])
                          n184 = Build Array (concatenate)(w795, w804) -> (w810:dbl[])
                          n185 = Bundle(w816, w814) -> (→"PhaseA-T":cluster{dbl[], dbl[]})  [unwired: 1 in]
                          n186 = Bundle(w822, w810) -> (→"Phaseh1-T":cluster{dbl[], dbl[]})  [unwired: 1 in]
                        }
                        frame #3 {
                          n187 = Wait (ms)(milliseconds to wait=u32 50) -> ()  [unwired: 1 out]
                        }
                      }
                    }
                  }
                  n188 = case shown="True" w565 {
                    tunnel: w568 -> [_ w600]
                    tunnel: w566 -> [_ w605]
                    tunnel: w567 -> [_ w603]
                    tunnel: w569 -> [_ w599]
                    tunnel: w570 -> [_ w598]
                    tunnel: w571 -> [_ w597]
                    frame False {
                    }
                    frame True {
                      n189 = Build Array(w605, w600, w599, w598, w597) -> (w602:dbl[])
                      n190 = call-poly <vilib>:"Write Delimited Spreadsheet.vi"("file path (dialog if empty)"=w603, "format (%.3f)"="%.10f", "1D data"=w602, "append to file? (new file:F)"=TRUE) -> ()  [unwired: 10 in, 2 out]
                    }
                  }
                }
              }
            }
          }
        }
      }
    }
    frame #2 {
      n191 = case shown="False" "Initialize" {
        tunnel: w840 -> [w841 w844]
        tunnel: w839 -> [w842 w843]
        frame False {
          n192 = Close Reference(reference=w842, error in (no error)=w841) -> ()  [unwired: 1 out]
        }
        frame True {
          w850 = 0 items=["Linear", "NoOvershoot", "Oscillate"] ("Approach")
          w851 = 0 items=["Persistent", "Driven"] ("Mode")
          w847 = 0 items=["FastSettle", "NoOvershoot"] ("Approach")
          n193 = call "SetTemperature.vi"("Approach"=w847, "Rate"=20.0, "Temperature"=2.0, "error in (no error)"=w844, "Instrument Ref In"=w843) -> ("error out"=w855:errorcluster, "Instrument Ref Out"=w854:refnum<k24>)  [unwired: 2 in, 1 out]
          n194 = call "SetField.vi"("Mode"=w851, "Approach"=w850, "Rate"=200.0, "Field"=0.0, "error in (no error)"=w855, "Instrument Ref In"=w854) -> ("error out"=w852:errorcluster, "Instrument Ref Out"=w853:refnum<k24>)  [unwired: 1 in, 1 out]
          n195 = Close Reference(reference=w853, error in (no error)=w852) -> ()  [unwired: 1 out]
        }
      }
    }
    frame #3 {
    }
  }
  n196 = case shown="True" "Read Status" {
    tunnel: w5 -> [_ w859]
    tunnel: w4 -> [_ w858]
    tunnel: w2 -> [_ w857]
    frame False {
    }
    frame True {
      n197 = while {
        tunnel: w859 -> [w862]
        tunnel: w858 -> [w861]
        tunnel: w857 -> [w860]
        stop <- w860 stop-if-true
        n198 = for {
          N: 10 -> [_]
          shift-right: [w877] -> _
          shift-left: w861 -> [w879]
          tunnel: w862 -> [w876]
          tunnel: [w874] -> _
          tunnel: [w871] -> w868
          tunnel: [w870] -> w867
          tunnel: [w872] -> w865 mode=indexing
          tunnel: [w873] -> w866 mode=indexing
          n199 = call "GetTemperature.vi"("error in (no error)"=w879, "Instrument Ref In"=w876) -> ("Temperature\nStatus"=w870:i32, "Temperature"=w873:dbl, "error out"=w878:errorcluster, "Instrument Ref Out"=w875:refnum<k24>)  [unwired: 3 in, 1 out]
          n200 = Wait (ms)(milliseconds to wait=u32 200) -> ()  [unwired: 1 out]
          n201 = call "GetField.vi"("error in (no error)"=w878, "Instrument Ref In"=w875) -> ("Field\nStatus"=w871:i32, "Field"=w872:dbl, "error out"=w877:errorcluster, "Instrument Ref Out"=w874:refnum<k24>)  [unwired: 3 in, 1 out]
        }
        "Field Status" <- w868
        "Temperature Status" <- w867
        n202 = call-poly <vilib>:"Mean.vi"("X"=w865) -> ("mean"=→"Field":dbl)  [unwired: 1 out]
        n203 = call-poly <vilib>:"Mean.vi"("X"=w866) -> ("mean"=→"Temperature":dbl)  [unwired: 1 out]
      }
    }
  }
